vi "Execute Selected.vi"(8 "error in":errorcluster, 10 "LineToExecute":u32, 11 "MLTFNC in":refnum<class "MLTFNC.lvclass">) -> (0 "error out":errorcluster, 3 "MLTFNC out":refnum<class "MLTFNC.lvclass">)   [LabVIEW 2019]
uses:
  Library/MLTFNC.lvclass
  C:/Users/Public/Documents/Development/builds/Instruments/Instruments.lvlibp/Library/Instruments.lvclass
  C:/Users/Public/Documents/Development/builds/Tools/Config.lvlibp/Config.lvclass
  C:/Users/Public/Documents/Development/builds/Engine/Engine.lvlibp/Project/Engine.lvclass
  C:/Users/Public/Documents/Development/builds/Engine/State Actor.lvlibp/Library/State Actor.lvclass
  C:/Users/Public/Documents/Development/builds/Engine/Panel Manager.lvlibp/Panel Actor/Panel Actor.lvclass
  C:/Users/Public/Documents/Development/builds/Engine/Monitored Actor.lvlibp/Monitored Actor/Monitored Actor/Monitored Actor.lvclass
  C:/Users/Public/Documents/Development/builds/Engine/Actor Framework.lvlibp/1abvi3w/vi.lib/ActorFramework/Actor/Actor.lvclass
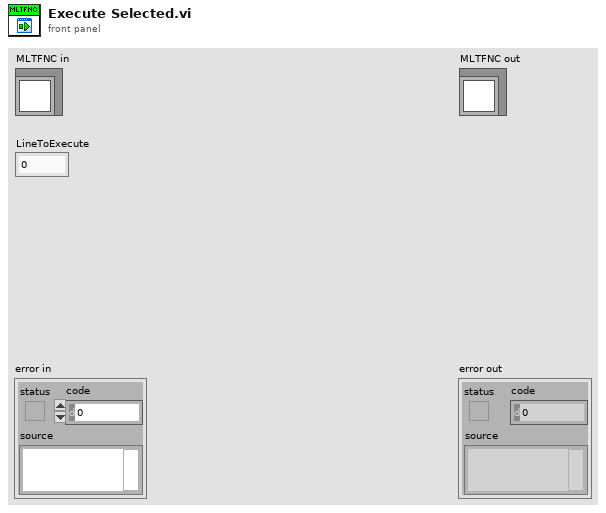
[diagram p1: front panel]
types:
  T1 = cluster{"Target":string, "Destination":string, "Action":string}
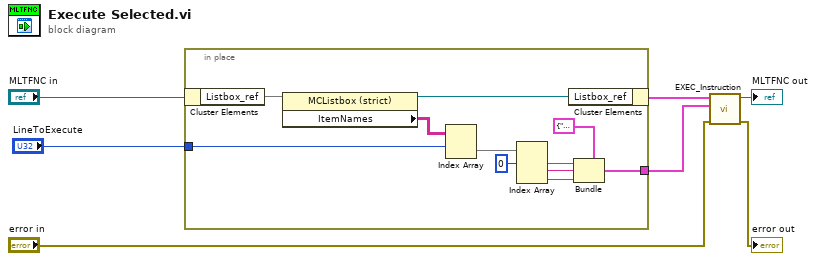
[diagram p0: block diagram]
diagram:
  n1 = in-place {
    in-place-border: "LineToExecute" -> [w15]
    in-place-border: [w9] -> w4
    n2 = in-place-cluster #1("MLTFNC in") -> ("Listbox_ref"=w18)
    n3 = property class="MCListbox (strict)"(reference=w18) -> (reference out=w17:refnum<vi>, "ItemNames"=w16:string[][])  [unwired: 1 in, 1 out]
    n4 = Index Array(array=w16, index (row)=w15) -> (element=w14:string[])  [unwired: 1 in]
    n5 = Index Array(array=w14, index #1=0 ("index")) -> (element #1=w12:string, element #2=w11:string, element #3=w10:string)  [unwired: 2 in]
    n6 = in-place-cluster #1("Listbox_ref"=w17) -> (w5:cluster{})
    n7 = Bundle(cluster=T1 {"Target"="", "Destination"="", "Action"=""} ("Instructions"), "Target"=w12, "Destination"=w11, "Action"=w10) -> (w9:T1)
  }
  n8 = call-dynamic "EXEC_Instruction.vi"("error in"="error in", "Instructions"=w4, "MLTFNC in"=w5) -> ("error out"=→"error out":errorcluster, "MLTFNC out"=→"MLTFNC out":refnum<class "MLTFNC.lvclass">)  [unwired: 7 in]
